vi "FV-get_water_values.vi"(7 "deg":dbl=22.5) -> (2 "Water Raw":T1 {"Sigma"."Data" format="%_9g"}, 6 "coerced temp":dbl)   [LabVIEW 2020, in "FV-file_viewer.lvlib"]
uses:
  FV-file_viewer.lvlib
  FV-water_cluster.ctl
  FV-single_XY_plot.ctl
panel:
  out "Sigma":cluster{"Array":dbl[], "Array":dbl[]}
  out "Epsilon":cluster{"Array":dbl[], "Array":dbl[]}
  out "20":dbl
  out "25":dbl
  out "Graph":cluster{"Frequency":dbl[], "S21_Imag":dbl[]}[](graph)
  out "string array 2":string[][](array[string])
  out "string array":string[](array[string])
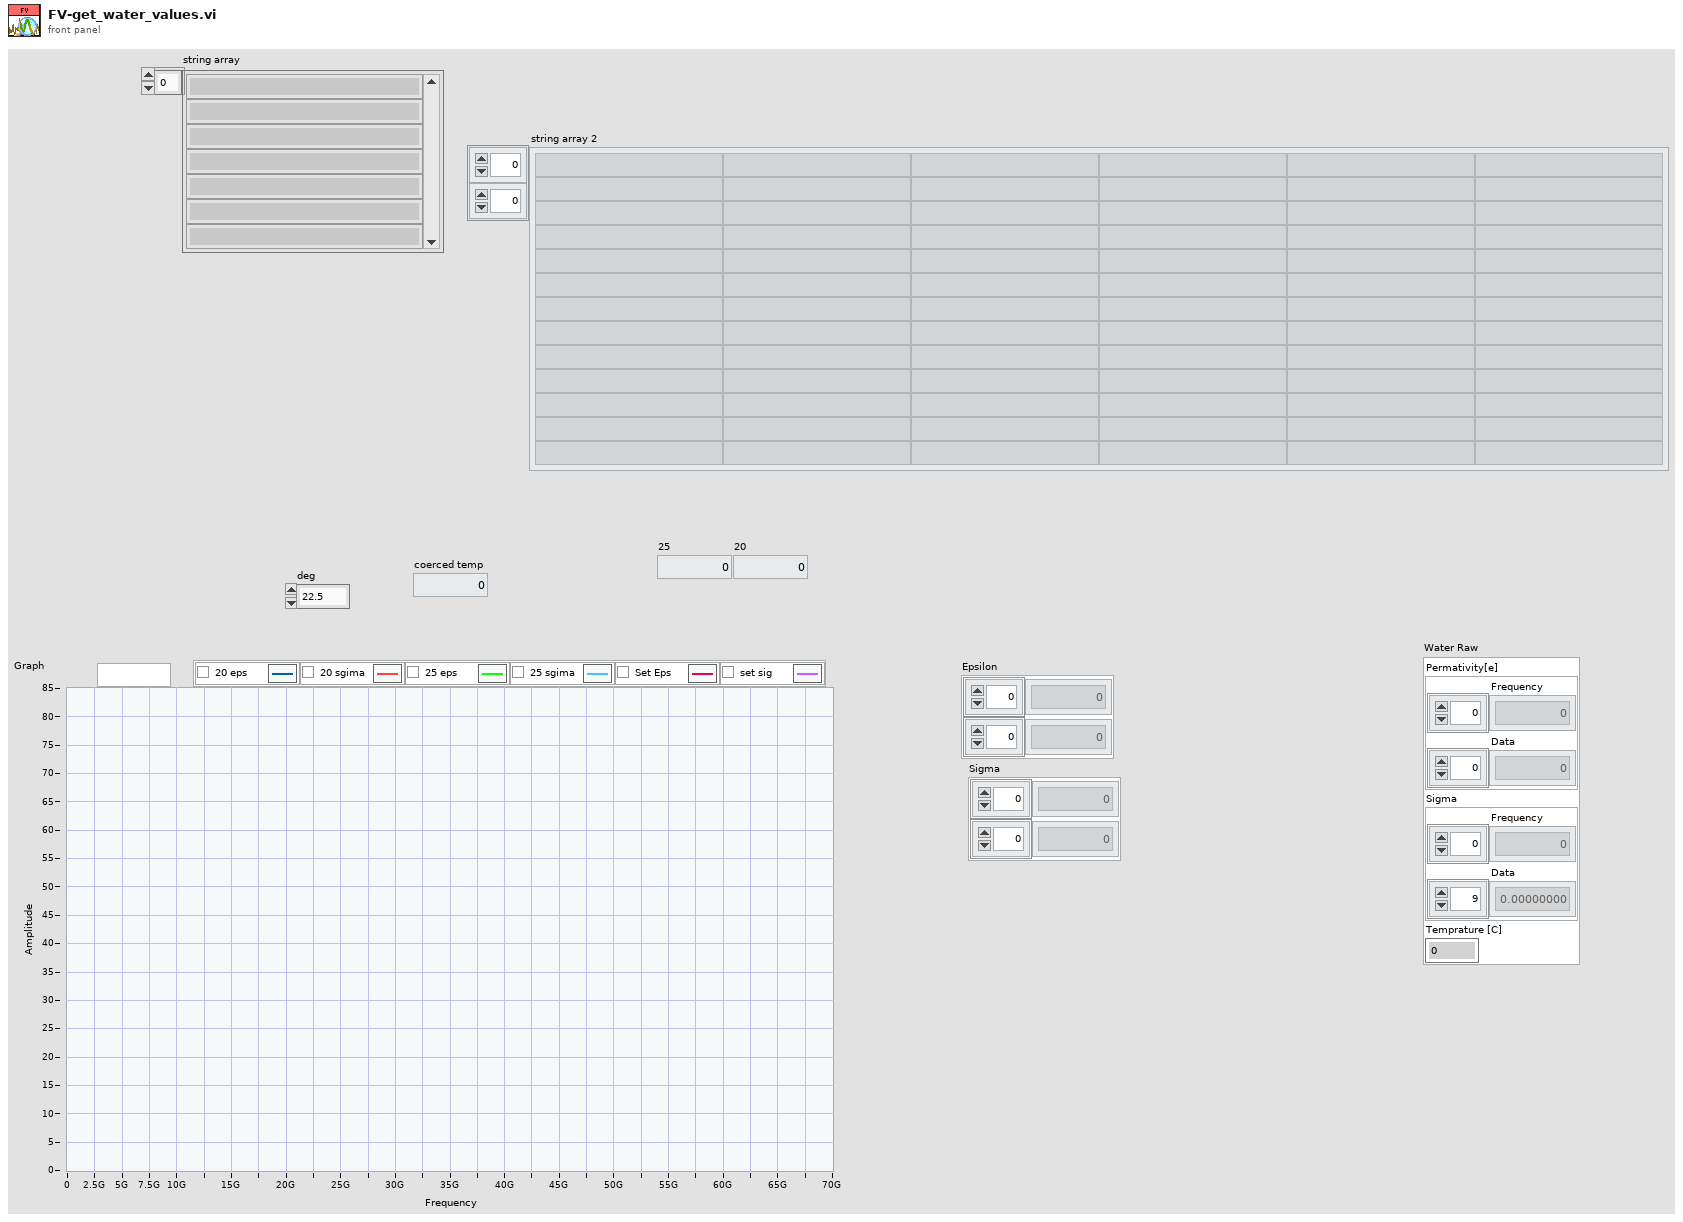
[diagram p1: front panel]
types:
  T1 = typedef "FV-file_viewer.lvlib/FV-water_cluster.ctl" = cluster{"Permativity[e]":T2, "Sigma":T2, "Temprature [C]":dbl}
  T2 = typedef "FV-file_viewer.lvlib/FV-single_XY_plot.ctl" = cluster{"Frequency":dbl[], "Data":dbl[]}
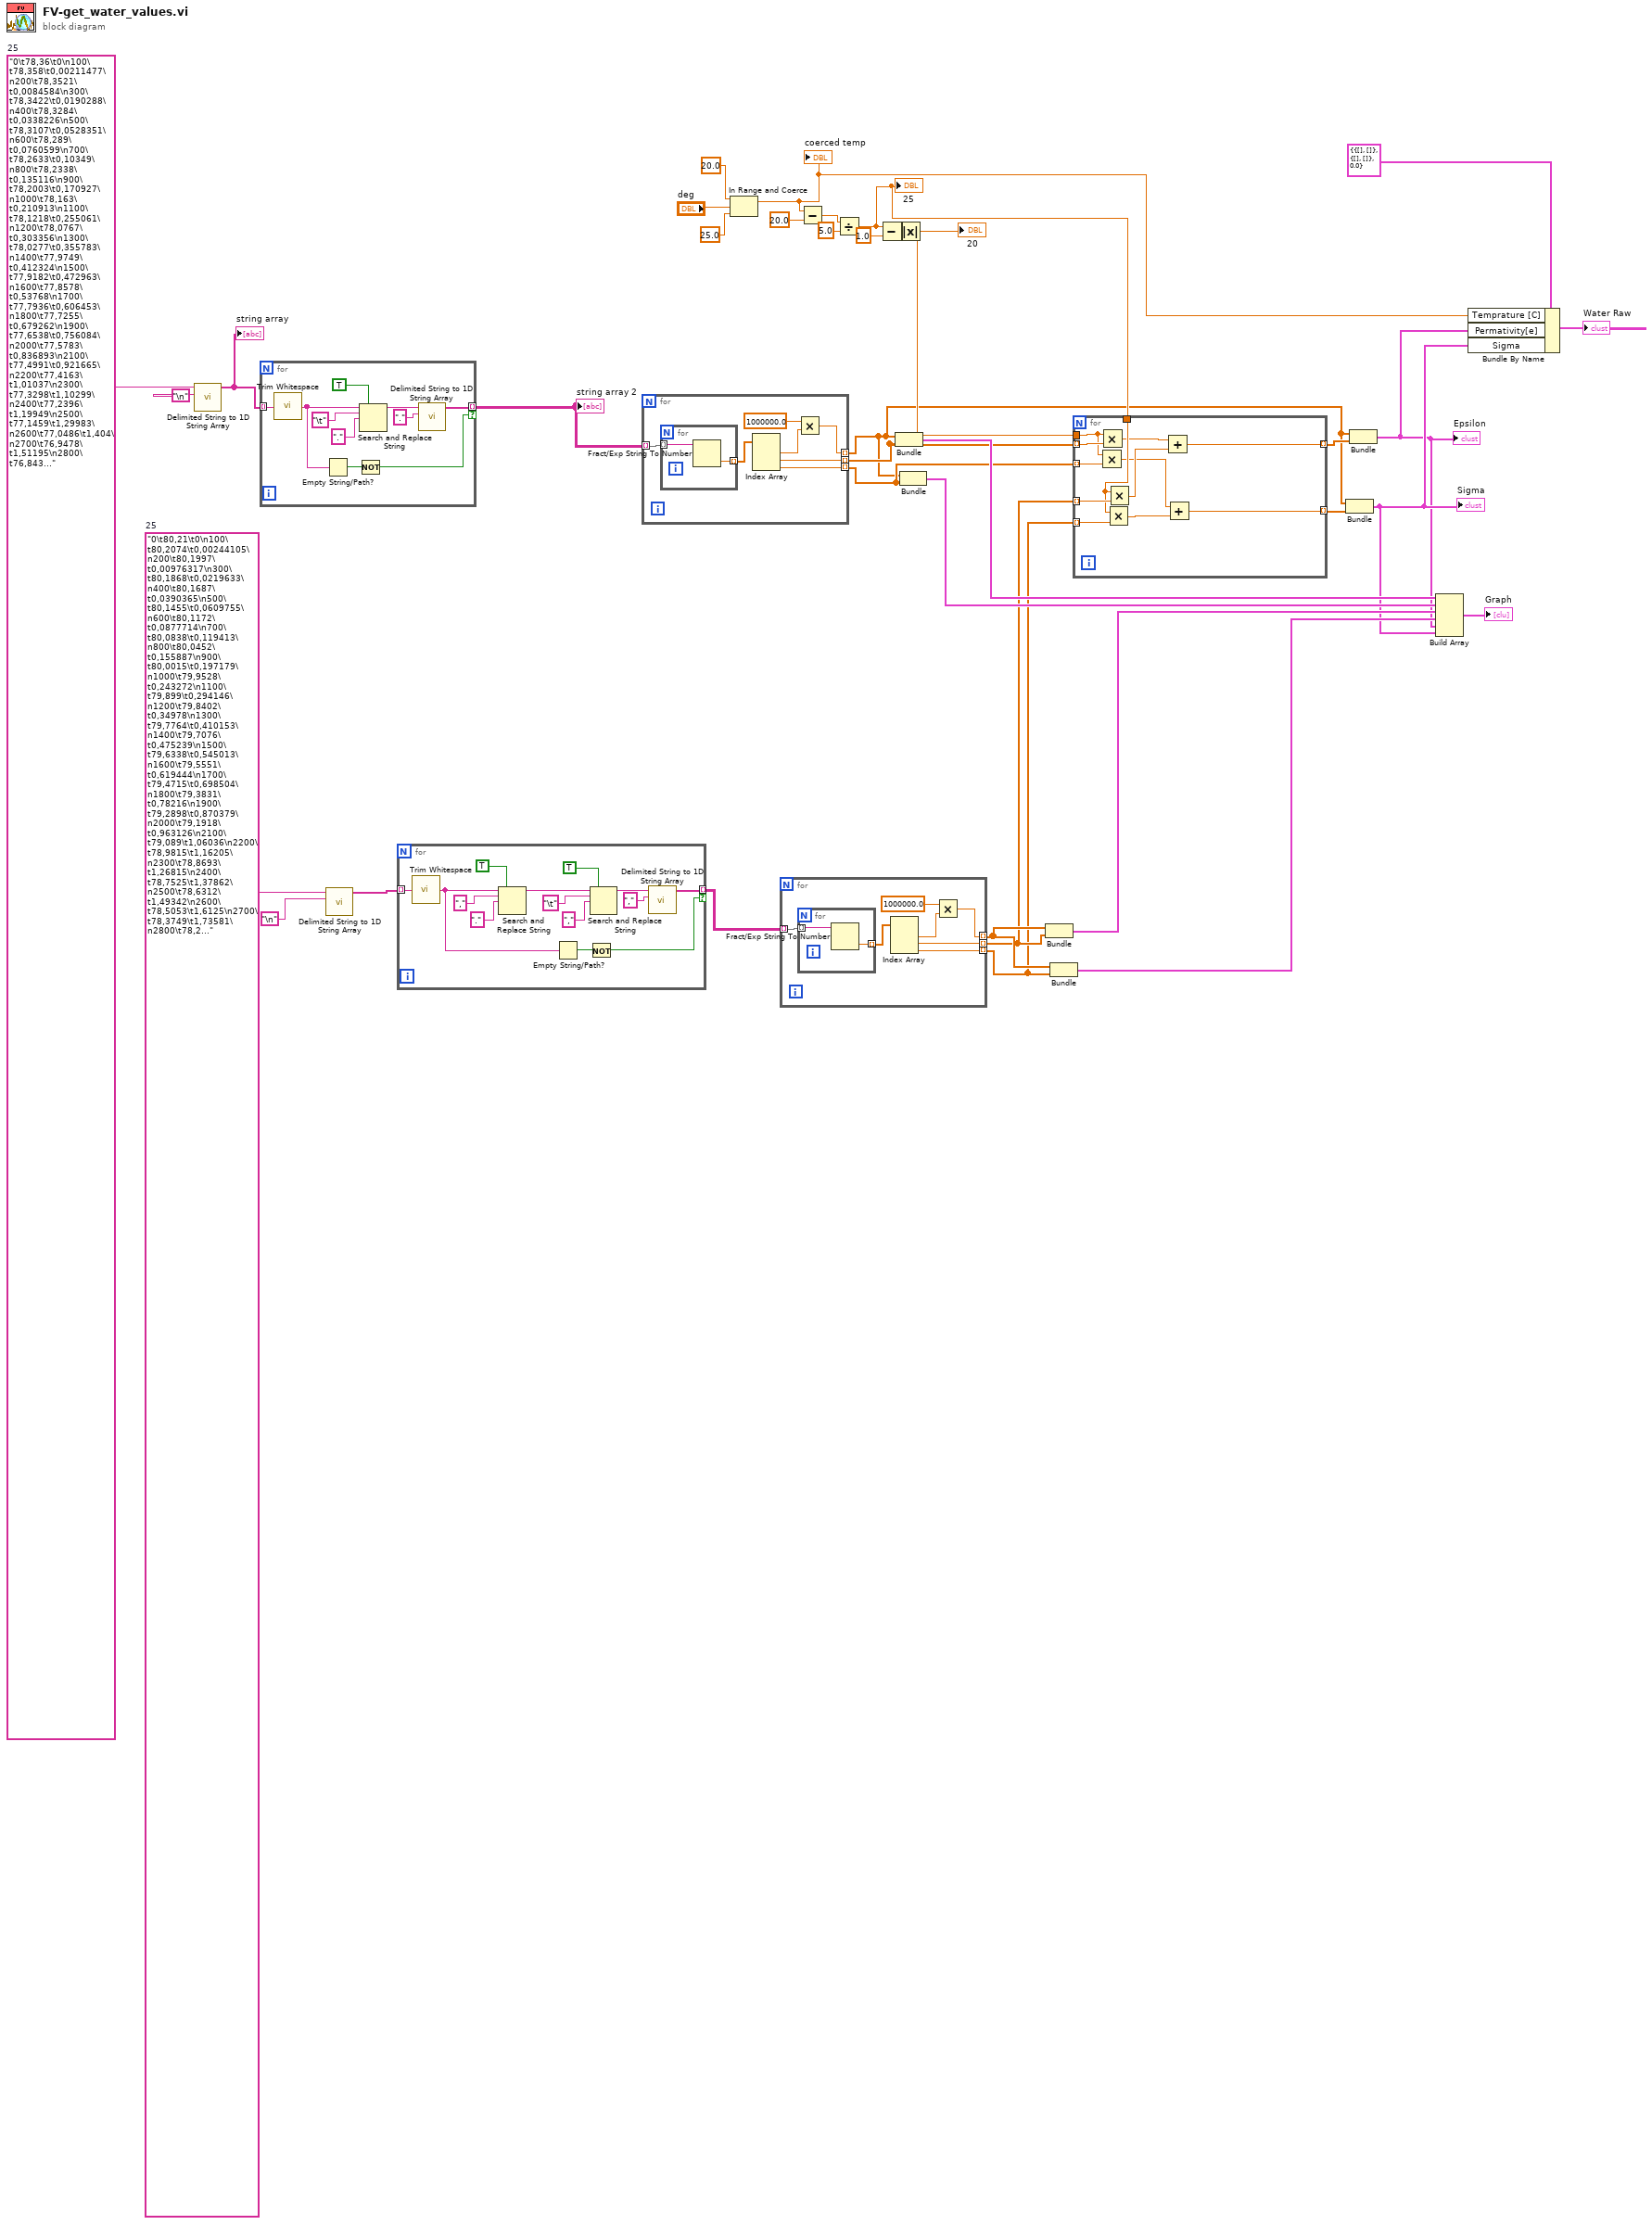
[diagram p0: block diagram]
diagram:
  w23 = "0\t80,21\t0\n100\t80,2074\t0,00244105\n200\t80,1997\t0,00976317\n300\t80,1868\t0,0219633\n400\t80,1687\t0,0390365\n500\t80,1455\t0,0609755\n600\t80,1172\t0,0877714\n700\t80,0838\t0,119413\n800\t80,0452\t0,155887\n900\t80,0015\t0,197179\n1000\t79,9528\t0,243272\n1100\t79,899\t0,294146\n1200\t79,8402\t0,34978\n1300\t79,7764\t0,410153\n1400\t79,7076\t0,475239\n1500\t79,6338\t0,545013\n1600\t79,5551\t0,619444\n1700\t79,4715\t0,698504\n1800\t79,3831\t0,78216\n1900\t79,2898\t0,870379\n2000\t79,1918\t0,963126\n2100\t79,089\t1,06036\n2200\t78,9815\t1,16205\n2300\t78,8693\t1,26815\n2400\t78,7525\t1,37862\n2500\t78,6312\t1,49342\n2600\t78,5053\t1,6125\n2700\t78,3749\t1,73581\n2800\t78,2401\t1,86332\n2900\t78,1009\t1,99496\n3000\t77,9574\t2,13069\n3100\t77,8097\t2,27045\n3200\t77,6577\t2,41421\n3300\t77,5016\t2,56189\n3400\t77,3414\t2,71345\n3500\t77,1771\t2,86882\n3600\t77,0089\t3,02797\n3700\t76,8367\t3,19081\n3800\t76,6607\t3,3573\n3900\t76,4809\t3,52738\n4000\t76,2973\t3,70098\n4100\t76,1101\t3,87805\n4200\t75,9194\t4,05852\n4300\t75,725\t4,24232\n4400\t75,5273\t4,42941\n4500\t75,3261\t4,6197\n4600\t75,1216\t4,81315\n4700\t74,9138\t5,00967\n4800\t74,7028\t5,20921\n4900\t74,4888\t5,41171\n5000\t74,2716\t5,61709\n5100\t74,0515\t5,82529\n5200\t73,8285\t6,03624\n5300\t73,6027\t6,24988\n5400\t73,374\t6,46613\n5500\t73,1427\t6,68494\n5600\t72,9088\t6,90624\n5700\t72,6723\t7,12995\n5800\t72,4333\t7,35601\n5900\t72,1919\t7,58436\n6000\t71,9481\t7,81493\n7000\t69,397\t10,228\n8000\t66,6869\t12,7915\n9000\t63,881\t15,4456\n10000\t61,0351\t18,1375\n11000\t58,1964\t20,8226\n12000\t55,4033\t23,4647\n13000\t52,6854\t26,0355\n14000\t50,0647\t28,5144\n15000\t47,5565\t30,887\n16000\t45,1704\t33,1439\n17000\t42,9116\t35,2805\n18000\t40,7816\t37,2953\n19000\t38,7793\t39,1893\n20000\t36,9015\t40,9655\n21000\t35,1437\t42,6282\n22000\t33,5005\t44,1825\n23000\t31,9658\t45,6342\n24000\t30,5334\t46,9891\n25000\t29,1968\t48,2533\n26000\t27,9499\t49,4328\n27000\t26,7864\t50,5334\n28000\t25,7005\t51,5605\n29000\t24,6867\t52,5195\n30000\t23,7397\t53,4153\n31000\t22,8545\t54,2525\n32000\t22,0267\t55,0356\n33000\t21,2519\t55,7684\n34000\t20,5262\t56,4549\n35000\t19,846\t57,0983\n36000\t19,2079\t57,7019\n37000\t18,6088\t58,2685\n38000\t18,0458\t58,801\n39000\t17,5164\t59,3018\n40000\t17,0181\t59,7732\n41000\t16,5486\t60,2173\n42000\t16,106\t60,6359\n43000\t15,6883\t61,031\n44000\t15,2939\t61,4041\n45000\t14,9211\t61,7568\n46000\t14,5684\t62,0904\n47000\t14,2345\t62,4062\n48000\t13,9182\t62,7054\n49000\t13,6182\t62,9891\n50000\t13,3336\t63,2583\n51000\t13,0634\t63,514\n52000\t12,8065\t63,7569\n53000\t12,5623\t63,9879\n54000\t12,3299\t64,2078\n55000\t12,1085\t64,4171\n56000\t11,8976\t64,6167\n57000\t11,6965\t64,8069\n58000\t11,5045\t64,9884\n59000\t11,3213\t65,1618\n60000\t11,1462\t65,3274\n61000\t10,9789\t65,4857\n62000\t10,8188\t65,6371\n63000\t10,6656\t65,782\n64000\t10,5189\t65,9208\n65000\t10,3783\t66,0537\n66000\t10,2436\t66,1812\n67000\t10,1143\t66,3035\n68000\t9,99028\t66,4208\n69000\t9,87118\t66,5334\n70000\t9,75677\t66,6417\n"  # 25
  w36 = "0\t78,36\t0\n100\t78,358\t0,00211477\n200\t78,3521\t0,0084584\n300\t78,3422\t0,0190288\n400\t78,3284\t0,0338226\n500\t78,3107\t0,0528351\n600\t78,289\t0,0760599\n700\t78,2633\t0,10349\n800\t78,2338\t0,135116\n900\t78,2003\t0,170927\n1000\t78,163\t0,210913\n1100\t78,1218\t0,255061\n1200\t78,0767\t0,303356\n1300\t78,0277\t0,355783\n1400\t77,9749\t0,412324\n1500\t77,9182\t0,472963\n1600\t77,8578\t0,53768\n1700\t77,7936\t0,606453\n1800\t77,7255\t0,679262\n1900\t77,6538\t0,756084\n2000\t77,5783\t0,836893\n2100\t77,4991\t0,921665\n2200\t77,4163\t1,01037\n2300\t77,3298\t1,10299\n2400\t77,2396\t1,19949\n2500\t77,1459\t1,29983\n2600\t77,0486\t1,404\n2700\t76,9478\t1,51195\n2800\t76,8435\t1,62366\n2900\t76,7356\t1,73908\n3000\t76,6244\t1,85819\n3100\t76,5097\t1,98095\n3200\t76,3917\t2,10732\n3300\t76,2703\t2,23727\n3400\t76,1456\t2,37075\n3500\t76,0177\t2,50772\n3600\t75,8865\t2,64815\n3700\t75,7522\t2,792\n3800\t75,6147\t2,93922\n3900\t75,4741\t3,08977\n4000\t75,3304\t3,2436\n4100\t75,1836\t3,40068\n4200\t75,0339\t3,56096\n4300\t74,8813\t3,72439\n4400\t74,7257\t3,89092\n4500\t74,5673\t4,06052\n4600\t74,4061\t4,23313\n4700\t74,2421\t4,40871\n4800\t74,0754\t4,5872\n4900\t73,906\t4,76857\n5000\t73,734\t4,95276\n5100\t73,5593\t5,13972\n5200\t73,3822\t5,32941\n5300\t73,2025\t5,52177\n5400\t73,0204\t5,71675\n5500\t72,8358\t5,91431\n5600\t72,649\t6,11438\n5700\t72,4598\t6,31694\n5800\t72,2683\t6,52191\n5900\t72,0746\t6,72926\n6000\t71,8788\t6,93892\n7000\t69,8118\t9,15187\n8000\t67,5806\t11,5407\n9000\t65,2312\t14,0561\n10000\t62,8063\t16,6522\n11000\t60,3443\t19,288\n12000\t57,8786\t21,9279\n13000\t55,4369\t24,5421\n14000\t53,042\t27,1061\n15000\t50,7116\t29,601\n16000\t48,4592\t32,0125\n17000\t46,2942\t34,3305\n18000\t44,2228\t36,5481\n19000\t42,2486\t38,6617\n20000\t40,3731\t40,6698\n21000\t38,5957\t42,5726\n22000\t36,9149\t44,3721\n23000\t35,3281\t46,0711\n24000\t33,8318\t47,673\n25000\t32,4223\t49,182\n26000\t31,0955\t50,6026\n27000\t29,8471\t51,9391\n28000\t28,6728\t53,1964\n29000\t27,5683\t54,3789\n30000\t26,5294\t55,4911\n31000\t25,5522\t56,5374\n32000\t24,6326\t57,5219\n33000\t23,7671\t58,4485\n34000\t22,9521\t59,3211\n35000\t22,1843\t60,1431\n36000\t21,4607\t60,9178\n37000\t20,7782\t61,6485\n38000\t20,1343\t62,3379\n39000\t19,5263\t62,9889\n40000\t18,9519\t63,6038\n41000\t18,4089\t64,1852\n42000\t17,8952\t64,7351\n43000\t17,409\t65,2557\n44000\t16,9484\t65,7487\n45000\t16,5119\t66,2161\n46000\t16,0979\t66,6593\n47000\t15,705\t67,08\n48000\t15,3318\t67,4795\n49000\t14,9772\t67,8592\n50000\t14,64\t68,2202\n51000\t14,3191\t68,5638\n52000\t14,0136\t68,8909\n53000\t13,7225\t69,2025\n54000\t13,445\t69,4996\n55000\t13,1804\t69,7829\n56000\t12,9277\t70,0534\n57000\t12,6865\t70,3117\n58000\t12,4559\t70,5585\n59000\t12,2355\t70,7945\n60000\t12,0246\t71,0203\n61000\t11,8228\t71,2364\n62000\t11,6295\t71,4433\n63000\t11,4443\t71,6416\n64000\t11,2667\t71,8317\n65000\t11,0964\t72,014\n66000\t10,933\t72,189\n67000\t10,7761\t72,357\n68000\t10,6254\t72,5184\n69000\t10,4805\t72,6735\n70000\t10,3412\t72,8226\n"  # 25
  n1 = call <vilib>:"Delimited String to 1D String Array.vi"("delimiter"="\n", "delimited string"=w36) -> ("string array"=w34:string[])  [unwired: 9 in]
  "string array" <- w34
  n2 = for {
    tunnel: w34 -> [w46] mode=indexing
    tunnel: [w45] -> w33 mode=indexing if=w37
    n3 = call <vilib>:"Trim Whitespace.vi"("string"=w46) -> ("trimmed string"=w39:string)  [unwired: 1 in]
    n4 = Empty String/Path?(string/path=w39) -> (empty?=w38:bool)
    n5 = Not(x=w38) -> (.not. x?=w37:bool)
    n6 = Search and Replace String(replace all?=TRUE ("replace all? (F)"), input string=w39, search string="\t", replace string="." ("replace string (\"\")")) -> (result string=w40:string)  [unwired: 4 in, 3 out]
    n7 = call <vilib>:"Delimited String to 1D String Array.vi"("delimiter"=".", "delimited string"=w40) -> ("string array"=w45:string[])  [unwired: 9 in]
  }
  "string array 2" <- w33
  n8 = call <vilib>:"Delimited String to 1D String Array.vi"("delimiter"="\n", "delimited string"=w23) -> ("string array"=w28:string[])  [unwired: 9 in]
  n9 = for {
    tunnel: w28 -> [w60] mode=indexing
    tunnel: [w59] -> w27 mode=indexing if=w52
    n10 = call <vilib>:"Trim Whitespace.vi"("string"=w60) -> ("trimmed string"=w49:string)  [unwired: 1 in]
    n11 = Search and Replace String(replace all?=TRUE ("replace all? (F)"), input string=w49, search string=",", replace string="." ("replace string (\"\")")) -> (result string=w48:string)  [unwired: 4 in, 3 out]
    n12 = Empty String/Path?(string/path=w49) -> (empty?=w53:bool)
    n13 = Not(x=w53) -> (.not. x?=w52:bool)
    n14 = Search and Replace String(replace all?=TRUE ("replace all? (F)"), input string=w48, search string="\t", replace string="," ("replace string (\"\")")) -> (result string=w54:string)  [unwired: 4 in, 3 out]
    n15 = call <vilib>:"Delimited String to 1D String Array.vi"("delimiter"=",", "delimited string"=w54) -> ("string array"=w59:string[])  [unwired: 9 in]
  }
  n16 = for {
    tunnel: w33 -> [w67] mode=indexing
    tunnel: [w62] -> w6 mode=indexing
    tunnel: [w65] -> w14 mode=indexing
    tunnel: [w64] -> w13 mode=indexing
    n17 = for {
      tunnel: w67 -> [w69] mode=indexing
      tunnel: [w68] -> w66 mode=indexing
      n18 = Fract/Exp String To Number(string=w69) -> (number=w68:dbl)  [unwired: 3 in, 1 out]
    }
    n19 = Index Array(array=w66) -> (element #1=w63:dbl, element #2=w65:dbl, element #3=w64:dbl)  [unwired: 3 in]
    n20 = Multiply(x=1000000.0, y=w63) -> (x*y=w62:dbl)
  }
  n21 = In Range and Coerce(upper limit=20.0, x="deg", lower limit=25.0) -> (coerced(x)=w3:dbl)  [unwired: 1 out]
  "coerced temp" <- w3
  n22 = for {
    tunnel: w27 -> [w76] mode=indexing
    tunnel: [w71] -> w26 mode=indexing
    tunnel: [w74] -> w12 mode=indexing
    tunnel: [w73] -> w11 mode=indexing
    n23 = for {
      tunnel: w76 -> [w78] mode=indexing
      tunnel: [w77] -> w75 mode=indexing
      n24 = Fract/Exp String To Number(string=w78) -> (number=w77:dbl)  [unwired: 3 in, 1 out]
    }
    n25 = Index Array(array=w75) -> (element #1=w72:dbl, element #2=w74:dbl, element #3=w73:dbl)  [unwired: 3 in]
    n26 = Multiply(x=1000000.0, y=w72) -> (x*y=w71:dbl)
  }
  n27 = Subtract(x=w3, y=20.0) -> (x-y=w18:dbl)
  n28 = Divide(x=w18, y=5.0) -> (x/y=w9:dbl)
  "25" <- w9
  n29 = Subtract(x=w9, y=1.0) -> (x-y=w15:dbl)
  n30 = Bundle(w6, w14) -> (w32:cluster{dbl[], dbl[]})  [unwired: 1 in]
  n31 = Absolute Value(x=w15) -> (abs(x)=w10:dbl)
  "20" <- w10
  n32 = Bundle(w6, w13) -> (w31:cluster{dbl[], dbl[]})  [unwired: 1 in]
  n33 = Bundle(w26, w12) -> (w25:cluster{dbl[], dbl[]})  [unwired: 1 in]
  n34 = Bundle(w26, w11) -> (w24:cluster{dbl[], dbl[]})  [unwired: 1 in]
  n35 = for {
    tunnel: w14 -> [w90] mode=indexing
    tunnel: w13 -> [w88] mode=indexing
    tunnel: w12 -> [w87] mode=indexing
    tunnel: w11 -> [w86] mode=indexing
    tunnel: w10 -> [w89]
    tunnel: w9 -> [w85]
    tunnel: [w80] -> w7 mode=indexing
    tunnel: [w79] -> w8 mode=indexing
    n36 = Multiply(x=w89, y=w88) -> (x*y=w82:dbl)
    n37 = Multiply(x=w89, y=w90) -> (x*y=w84:dbl)
    n38 = Multiply(x=w85, y=w86) -> (x*y=w81:dbl)
    n39 = Multiply(x=w85, y=w87) -> (x*y=w83:dbl)
    n40 = Add(x=w84, y=w83) -> (x+y=w80:dbl)
    n41 = Add(x=w82, y=w81) -> (x+y=w79:dbl)
  }
  n42 = Bundle(w6, w8) -> (w2:cluster{dbl[], dbl[]})  [unwired: 1 in]
  "Sigma" <- w2
  n43 = Bundle(w6, w7) -> (w1:cluster{dbl[], dbl[]})  [unwired: 1 in]
  "Epsilon" <- w1
  n44 = Build Array(w32, w31, w25, w24, w1, w2) -> (→"Graph":cluster{dbl[], dbl[]}[])
  n45 = Bundle By Name(cluster=T1 {"Permativity[e]"={"Frequency"=[], "Data"=[]}, "Sigma"={"Frequency"=[], "Data"=[]}, "Temprature [C]"=0.0} ("Water Raw"), "Temprature [C]"=w3, "Permativity[e]"=w1, "Sigma"=w2) -> (→"Water Raw":T1)
